vi "CE14. Read_kW(subVI).vi"(8 "error in (no error)":errorcluster, 9 "milliseconds to wait(200)":u32=200, 11 "VISA resource name":refnum<visa-resource-name>) -> (0 "error out":errorcluster, 1 "data out":T1, 2 "read buffer":string, 3 "VISA resource name out":refnum<visa-resource-name>)   [LabVIEW 2018, in "CE14_eMIC.lvlib"]
uses:
  CE14_eMIC.lvlib
  type defs/CE14.data.ctl
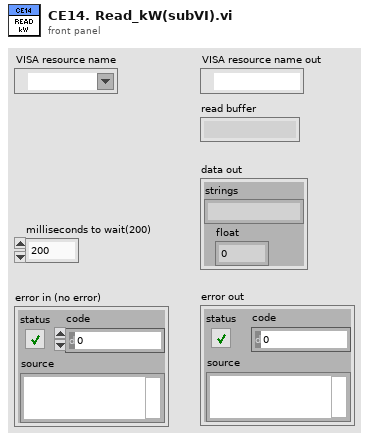
[diagram p1: front panel]
types:
  T1 = typedef "CE14_eMIC.lvlib/CE14.data.ctl" = cluster{"strings":string, "float":dbl}
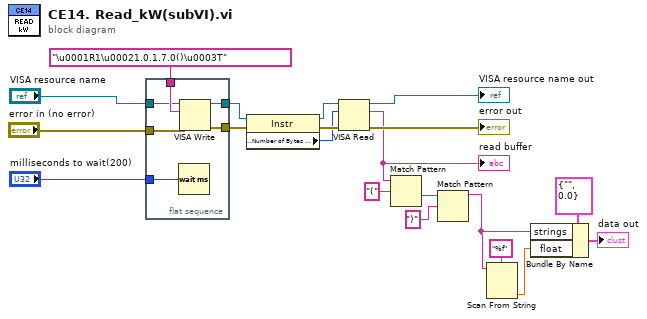
[diagram p0: block diagram]
diagram:
  n1 = flat-sequence {
    tunnel: "\u0001R1\u00021.0.1.7.0()\u0003T" -> [w26]
    tunnel: "VISA resource name" -> [w25]
    tunnel: "error in (no error)" -> [w24]
    tunnel: [w23] -> w17
    tunnel: [w22] -> w16
    tunnel: "milliseconds to wait(200)" -> [w21]
    frame #0 {
      n2 = Wait (ms)(milliseconds to wait=w21) -> ()  [unwired: 1 out]
      n3 = VISA Write(VISA resource name=w25, write buffer=w26, error in (no error)=w24) -> (VISA resource name out=w22:refnum<visa-resource-name>, error out=w23:errorcluster)  [unwired: 1 out]
    }
  }
  n4 = property class="Instr"(reference=w16, error in=w17) -> (reference out=w13:refnum<visa-resource-name>, error out=w15:errorcluster, "Serial Settings:Number of Bytes at Serial Port"=w14:u32)
  n5 = VISA Read(VISA resource name=w13, byte count=w14, error in (no error)=w15) -> (VISA resource name out=→"VISA resource name out":refnum<visa-resource-name>, read buffer=w9:string, error out=→"error out":errorcluster)  [unwired: 1 out]
  "read buffer" <- w9
  n6 = Match Pattern(string=w9, regular expression="(") -> (after substring=w7:string)  [unwired: 1 in, 3 out]
  n7 = Match Pattern(string=w7, regular expression=")") -> (before substring=w3:string)  [unwired: 1 in, 3 out]
  n8 = Scan From String(format string="%f", input string=w3) -> (output 1=w2:dbl)  [unwired: 3 in, 3 out]
  n9 = Bundle By Name(cluster=T1 {"strings"="", "float"=0.0} ("CE14. Data"), "strings"=w3, "float"=w2) -> (→"data out":T1)
